vi "memory_load_MLP_3_C_1.vi"() -> ()   [LabVIEW 2020]
panel:
  out "text":string
  out "array":dbl[](array[numeric])
  out "appended path":path
  out "Array":fxp<+/-,32,16>[](array[numeric])
  out "Init Data Out":fxp<+/-,32,16>[][](array[numeric])
  out "size(s)":i32
  # "For Initialization VI requirements and help, please read directions located on Block Diagram."
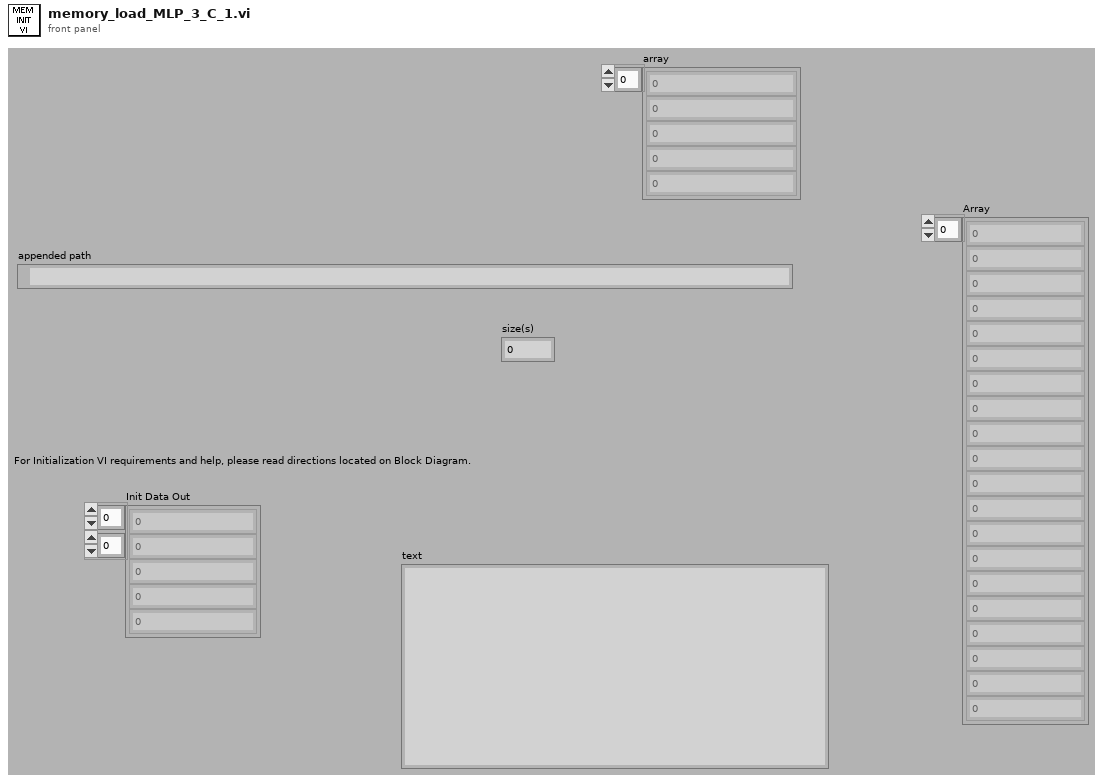
[diagram p1: front panel]
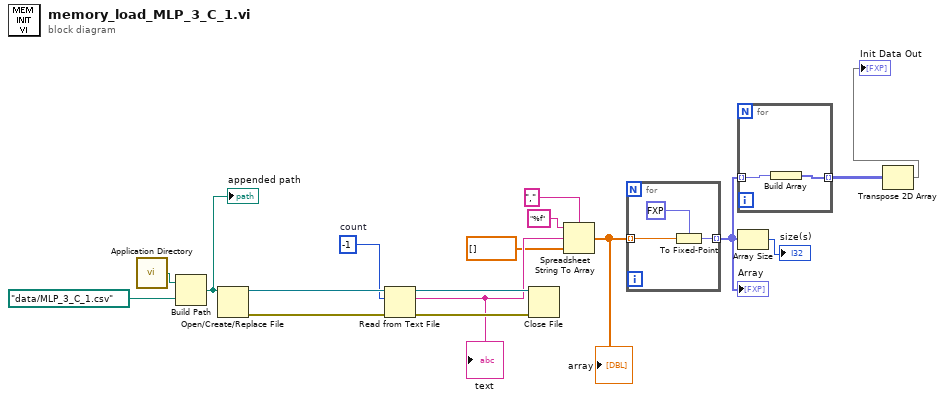
[diagram p0: block diagram]
diagram:
  w6 = -1  # count
  n1 = call <vilib>:"Application Directory.vi"() -> ("Application Directory"=w10:path)
  n2 = Build Path(base path=w10, name or relative path=path "data/MLP_3_C_1.csv" ("default name")) -> (appended path=w9:path)
  "appended path" <- w9
  n3 = Open/Create/Replace File(file path (use dialog)=w9) -> (refnum out=w14:refnum<file>, error out=w15:errorcluster)  [unwired: 5 in, 1 out]
  n4 = Read from Text File(file (use dialog)=w14, count=w6, error in=w15) -> (refnum out=w13:refnum<file>, text=w11:string, error out=w12:errorcluster)  [unwired: 1 in, 1 out]
  "text" <- w11
  n5 = Close File(refnum=w13, error in=w12) -> ()  [unwired: 2 out]
  n6 = Spreadsheet String To Array(delimiter (Tab)=",", format string="%f", spreadsheet string=w11, array type (2D Dbl)=dbl[] []) -> (array=w3:dbl[])
  "array" <- w3
  n7 = for {
    tunnel: w3 -> [w20] mode=indexing
    tunnel: [w19] -> w16 mode=indexing
    n8 = To Fixed-Point(fixed-point type=fxp<+/-,32,16> 0.0 ("fixed-point"), number=w20) -> (fixed-point=w19:fxp<+/-,32,16>)
  }
  "Array" <- w16
  n9 = for {
    tunnel: w16 -> [w22] mode=indexing
    tunnel: [w21] -> w2 mode=indexing
    n10 = Build Array(w22) -> (w21:fxp<+/-,32,16>[])
  }
  n11 = Array Size(array=w16) -> (size(s)=→"size(s)":i32)
  n12 = Transpose 2D Array(2D array=w2) -> (transposed array=→"Init Data Out":fxp<+/-,32,16>[][])
